vi "Kenbak-1.vi"() -> ()   [LabVIEW 2012]
uses:
  Blocks/NegJKflipFlop.vi
  <vilib>/Waveform/DTblOps.llb/DTbl Boolean Array to Digital.vi
panel:
  out "mem":u8 format="%x"
  in  "Set":bool
  in  "Oct":u8 format="%o"
  out "number":u32
  out "Array":bool[](array[boolean])
  in  "Loop":bool
  in  "Step 256":bool
  in  "Step 64":bool
  in  "Step 8":bool
  in  "Step 1":bool
  out "JS4":bool
  out "JS3":bool
  out "JS2":bool
  out "JS1":bool
  out "JS0":bool
  out "JDL1":bool
  out "JDL0":bool
  out "KP":bool
  out "PF":bool
  out "PT":bool
  out "PO":bool
  out "ED":bool
  out "WD":bool
  out "BM":bool
  out "WT":bool
  out "WL":bool
  out "WJ":bool
  out "WK":bool
  out "CY":bool
  out "OV":bool
  out "OF":bool
  out "CR":bool
  out "SUM":bool
  out "ADD":bool
  out "C":bool
  out "JC":bool
  out "TS":bool
  out "BD":bool
  out "B":bool
  out "A":bool
  out "LONGLOGIC":bool
  out "LS":bool
  out "RR":bool
  out "BT":bool
  out "TX":bool
  out "HF":bool
  out "JW3":bool
  out "JW7":bool
  out "W7":bool
  out "W6":bool
  out "W5":bool
  out "W4":bool
  out "W3":bool
  out "W2":bool
  out "W1":bool
  out "W0":bool
  out "K7":bool
  out "K6":bool
  out "K5":bool
  out "K4":bool
  out "K3":bool
  out "K2":bool
  out "K1":bool
  out "K0":bool
  out "KS":bool
  out "Run":bool
  out "Input":bool
  out "Mem":bool
  out "Add":bool
  out "X4":bool
  out "X3":bool
  out "X2":bool
  out "X1":bool
  out "BU":bool
  in  "S7":bool
  in  "S6":bool
  in  "S5":bool
  in  "S4":bool
  in  "S3":bool
  in  "S2":bool
  in  "S1":bool
  in  "S0":bool
  out "MR":bool
  out "FT":bool
  out "I4":bool
  out "I5":bool
  out "I6":bool
  out "I7":bool
  out "I3":bool
  out "I2":bool
  out "I1":bool
  out "I0":bool
  out "CL":bool
  out "DA":bool
  out "HT":bool
  out "EA":bool
  out "DD":bool
  out "EN":bool
  out "GO":bool
  out "UT":bool
  out "IN":bool
  in  "Clear":bool
  in  "Disp\nAdd":bool
  in  "Stop":bool
  in  "Set\nAdd":bool
  in  "Read\nMem":bool
  in  "Store\nMem":bool
  in  "Start":bool
  out "R":bool
  out "A7":bool
  out "SQ":bool
  out "SP":bool
  out "SW":bool
  out "SC":bool
  out "SD":bool
  out "SZ":bool
  out "SG":bool
  out "SM":bool
  out "SH":bool
  out "SK":bool
  out "SF":bool
  out "SN":bool
  out "SJ":bool
  out "SL":bool
  out "SA":bool
  out "QB":bool
  out "SX":bool
  out "SY":bool
  out "SB":bool
  out "ST":bool
  out "SV":bool
  out "SE":bool
  out "SU":bool
  out "SS":bool
  out "SR":bool
  out "QE":bool
  out "QF":bool
  out "QD":bool
  out "QC":bool
  in  "Plot?":bool
  out "Carry?":bool
  out "/ T7 \\":bool
  out "MemLoc":u8
  in  "Wait":u32=50
  in  "Diag?":bool
  out "LC":bool
  out "CM":bool
  out "L7":bool
  out "L6":bool
  out "L5":bool
  out "L4":bool
  out "L3":bool
  out "L2":bool
  out "L1":bool
  out "L0":bool
  out "Sigs":digitaldata(graph)
  out "T7":bool
  out "T6":bool
  out "T5":bool
  out "T4":bool
  out "T3":bool
  out "T2":bool
  out "T1":bool
  out "T0":bool
  out "F1":bool
  out "F2":bool
  out "C7":bool
  out "CP":bool
  out "CT":bool
  in  "Slices":u32=2
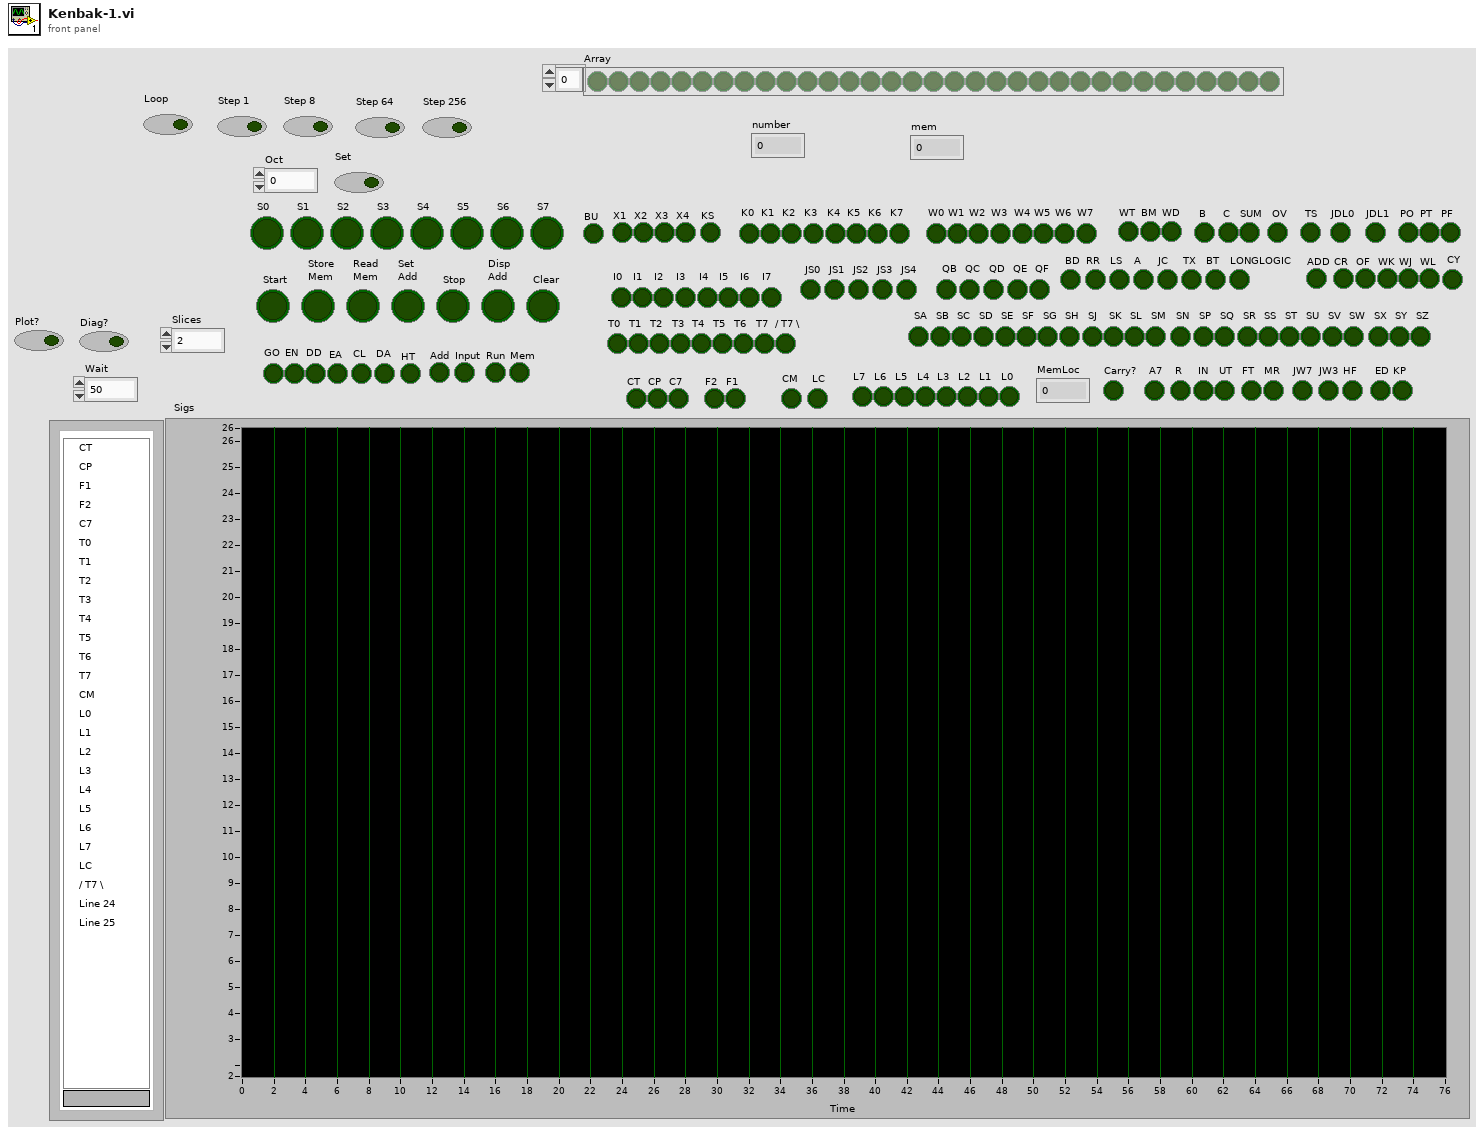
[diagram p1: front panel]
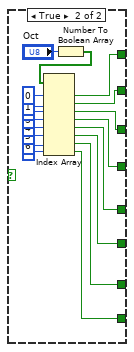
[diagram p2: hidden frame]
diagram:
  n1 = while {
    stop <- FALSE stop-if-true
    w68 = TRUE ("x")
    w107 = FALSE ("Serial\nInput")
    w149 = TRUE ("Set")
    w198 = TRUE ("Set")
    w199 = TRUE ("Set")
    w210 = FALSE ("y")
    w224 = TRUE ("Reset")
    w238 = TRUE ("Set")
    w249 = TRUE ("Set")
    w457 = TRUE ("Set")
    w458 = TRUE ("Set")
    w472 = TRUE ("Set")
    w605 = TRUE ("Set")
    w622 = TRUE ("Set")
    w629 = FALSE ("B")
    w630 = FALSE ("Mode\nControl")
    w633 = TRUE ("Set")
    w637 = FALSE ("B")
    w638 = FALSE ("Mode\nControl")
    w644 = TRUE
    w650 = TRUE ("Set")
    w652 = TRUE ("Set")
    # "JSX  0  1  2  3  4\nQB = 1, 0, 0, 1, 0\nQC = 0, 0, 0, 0, 0\nQD = 1, 0, 0, 0, 0\nQE = 1, 1, 0, 0, 0\nQF = 0, 1, 0, 0, 0\nSA = 0, 0, 0, 1, 0\nSB = 0, 0, 1, 1, 0\nSC = 0, 1, 0, 1, 1\nSD = 1, 1, 0, 1, 1\nSE = 1, 1, 1, 0, 0\nSF = 1, 1, 0, 0, 1\nSG = 1, 1, 1, 0, 1\nSH = 1, 0, 0, 0, 1\nSJ = 1, 0, 1, 0, 1\nSK = 0, 1, 0, 0, 1\nSL = 0, 1, 1, 0, 1\nSM = 0, 0, 0, 0, 1\nSN = 0, 0, 1, 0, 1\nSP = 0, 0, 0, 1, 1\nSQ = 0, 1, 1, 1, 1\nSR = 0, 0, 1, 0, 0\nSS = 1, 0, 1, 0, 0\nST = 1, 0, 1, 1, 0\nSU = 0, 1, 1, 0, 0\nSV = 0, 1, 1, 1, 0\nSW = 1, 0, 0, 1, 1\nSX = 0, 1, 0, 1, 0\nSY = 1, 1, 0, 1, 0\nSZ = 0, 0, 1, 1, 1"
    # "-IN+-BU"
    # "-IN+-CL"
    # "I11"
    # "I10"
    # "I2+-I1+I0"
    # "EN+DD"
    # "JS0"
    # "JS1"
    # "JS2"
    # "JS3"
    # "JS4"
    # "JS0B"
    # "JS0A"
    # "JS1B"
    # "JS2A"
    # "CM"
    # "JS1A"
    # "JS3A"
    # "JS3-4B"
    # "G5"
    # "G4"
    # "G3"
    # "G2"
    # "G1"
    n2 = call "Clock.vi"("Slices"="Slices") -> ("Clk"=w654:bool)  [unwired: 10 in]
    "CT" <- w654
    n3 = case shown="False" "Set" {
      tunnel: ["S0" w678] -> w44
      tunnel: ["S1" w669] -> w43
      tunnel: ["S2" w668] -> w41
      tunnel: ["S3" w667] -> w39
      tunnel: ["S4" w666] -> w37
      tunnel: ["S5" w665] -> w35
      tunnel: ["S6" w664] -> w33
      tunnel: ["S7" w663] -> w30
      frame False {
      }
      frame True {
        n4 = Number To Boolean Array(number="Oct") -> (Boolean array=w679:bool[])
        n5 = Index Array(array=w679, index #1=0 ("index"), index #2=1 ("index"), index #3=2 ("index"), index #4=3 ("index"), index #5=4 ("index"), index #6=5 ("index"), index #7=6 ("index"), index #8=7 ("index")) -> (element #1=w678:bool, element #2=w669:bool, element #3=w668:bool, element #4=w667:bool, element #5=w666:bool, element #6=w665:bool, element #7=w664:bool, element #8=w663:bool)
      }
    }
    n6 = Not And(1:w654, 2:w654) -> (0:w653:bool)
    n7 = feedback #1() -> (w651:bool)  [unwired: 1 in]
    n8 = call "DflipFlop.vi"("D"=w651, "Clock"=w653, "Reset"=w652, "Set"=w652) -> ("/Q\\"=w27:bool, "Q"=w639:bool)  [unwired: 6 in]
    n9 = feedback-in #1(w27) -> ()
    n10 = Not(x=w35) -> (.not. x?=w34:bool)
    n11 = Not(x=w33) -> (.not. x?=w32:bool)
    n12 = Not(x=w30) -> (.not. x?=w31:bool)
    n13 = Not(x=w44) -> (.not. x?=w45:bool)
    n14 = Not(x=w43) -> (.not. x?=w42:bool)
    n15 = Not(x=w41) -> (.not. x?=w40:bool)
    n16 = Not(x=w39) -> (.not. x?=w38:bool)
    n17 = Not(x=w37) -> (.not. x?=w36:bool)
    n18 = feedback #2() -> (w607:bool)  [unwired: 1 in]
    n19 = Not(x="Stop") -> (.not. x?=w4:bool)
    "HT" <- w4
    n20 = Not(x="Start") -> (.not. x?=w464:bool)
    n21 = Not(x="Read\nMem") -> (.not. x?=w462:bool)
    n22 = Not(x="Set\nAdd") -> (.not. x?=w461:bool)
    n23 = Not(x="Disp\nAdd") -> (.not. x?=w392:bool)
    "DA" <- w392
    n24 = Not(x="Clear") -> (.not. x?=w80:bool)
    "CL" <- w80
    n25 = Not(x="Store\nMem") -> (.not. x?=w463:bool)
    n26 = feedback #3() -> (w647:bool)  [unwired: 1 in]
    n27 = Compound Arithmetic op=AND(w647, w647, w607) -> (w649:bool)
    n28 = Not(x=w649) -> (.not. x?=w648:bool)
    n29 = call "DflipFlop.vi"("D"=w648, "Clock"=w639, "Reset"=w650, "Set"=w650) -> ("/Q\\"=w643:bool, "Q"=w642:bool)  [unwired: 6 in]
    n30 = feedback-in #3(w642) -> ()
    n31 = Not And(1:w639, 2:w639) -> (0:w641:bool)
    n32 = feedback #4() -> (w635:bool)  [unwired: 1 in]
    n33 = Not And(1:w635, 2:w639) -> (0:w640:bool)
    n34 = Not And(1:w635, 2:w635) -> (0:w606:bool)
    "/ T7 \\" <- w606
    n35 = feedback-in #2(w606) -> ()
    n36 = Not(x=w641) -> (.not. x?=w106:bool)
    "CP" <- w106
    n37 = call "7495.vi"("Clk 1\nR-Shift"=w106, "Serial\nInput"=w635, "Clk 2\nL-Shift"=w106, "Mode\nControl"=w638, "D"=w638, "C"=w638, "B"=w638, "A"=w638) -> ("OD"=w409:bool, "OC"=w410:bool, "OB"=w85:bool, "OA"=w87:bool)
    "T0" <- w87
    "T1" <- w85
    "T2" <- w410
    "T3" <- w409
    n38 = Not And(1:w45, 2:w87) -> (0:w406:bool)
    n39 = Not And(1:w42, 2:w85) -> (0:w405:bool)
    n40 = Not And(1:w40, 2:w410) -> (0:w404:bool)
    n41 = Not And(1:w38, 2:w409) -> (0:w403:bool)
    n42 = Not(x=w640) -> (.not. x?=w234:bool)
    "C7" <- w234
    n43 = Not And(1:w234, 2:w234) -> (0:w513:bool)
    n44 = call "7495.vi"("Clk 1\nR-Shift"=w106, "Serial\nInput"=FALSE ("Serial\nInput"), "Clk 2\nL-Shift"=w106, "Mode\nControl"=w409, "D"=w637, "C"=w637, "B"=w637, "A"=w409) -> ("OD"=w14:bool, "OC"=w407:bool, "OB"=w408:bool, "OA"=w296:bool)
    "T4" <- w296
    "T5" <- w408
    "T6" <- w407
    "T7" <- w14
    n45 = feedback-in #4(w14) -> ()
    n46 = Not And(1:w36, 2:w296) -> (0:w402:bool)
    n47 = Not And(1:w234, 2:w234) -> (0:w456:bool)
    n48 = feedback #5() -> (w394:bool)  [unwired: 1 in]
    n49 = feedback #6() -> (w393:bool)  [unwired: 1 in]
    n50 = Not And(1:w34, 2:w408) -> (0:w401:bool)
    n51 = Compound Arithmetic op=AND(w643, w644, w27) -> (w645:bool)
    n52 = Compound Arithmetic op=AND(w644, w27, w642) -> (w646:bool)
    n53 = Not(x=w645) -> (.not. x?=w73:bool)
    "F1" <- w73
    n54 = Not(x=w646) -> (.not. x?=w71:bool)
    "F2" <- w71
    n55 = feedback #7() -> (w455:bool)  [unwired: 1 in]
    n56 = call "DflipFlop.vi"("D"=w455, "Clock"=w456, "Reset"=w458, "Set"=w458) -> ("Q"=w378:bool)  [unwired: 6 in, 1 out]
    "UT" <- w378
    n57 = Not And(1:w32, 2:w407) -> (0:w400:bool)
    n58 = Exclusive Or(1:w106, 2:TRUE ("x")) -> (0:w621:bool)
    n59 = Not And(1:w31, 2:w14) -> (0:w399:bool)
    n60 = Compound Arithmetic op=AND(w80, w80, w80) -> (w82:bool)
    n61 = Not(x=w82) -> (.not. x?=w81:bool)
    n62 = Compound Arithmetic op=AND(w406, w405, w404, w403, w402, w401, w400, w399) -> (w25:bool)
    "BU" <- w25
    n63 = Not And(1:w25, 2:w25) -> (0:w26:bool)
    n64 = feedback #8() -> (w627:bool)  [unwired: 1 in]
    n65 = feedback #9() -> (w619:bool)  [unwired: 1 in]
    n66 = Not And(1:w619, 2:w627) -> (0:w632:bool)
    n67 = Not And(1:w606, 2:w632) -> (0:w631:bool)
    n68 = Exclusive Or(1:w619, 2:w627) -> (0:w628:bool)
    n69 = call "7495.vi"("Clk 1\nR-Shift"=w106, "Serial\nInput"=w628, "Clk 2\nL-Shift"=w106, "Mode\nControl"=w630, "D"=w630, "C"=w630, "A"=w619) -> ("OD"=w612:bool, "OC"=→"L5":bool, "OB"=→"L6":bool, "OA"=→"L7":bool)  [unwired: 1 in]
    "L4" <- w612
    n70 = call "DflipFlop.vi"("D"=w631, "Clock"=w621, "Reset"=w633, "Set"=w633) -> ("Q"=w451:bool)  [unwired: 6 in, 1 out]
    "LC" <- w451
    n71 = call "DflipFlop.vi"("D"=w451, "Clock"=w456, "Reset"=w457, "Set"=w457) -> ("Q"=w78:bool)  [unwired: 6 in, 1 out]
    "IN" <- w78
    n72 = call "7495.vi"("Clk 1\nR-Shift"=w78, "Serial\nInput"=FALSE ("Serial\nInput"), "Clk 2\nL-Shift"=w78, "Mode\nControl"=TRUE ("Mode\nControl"), "D"=w461, "C"=w462, "B"=w463, "A"=w464) -> ("OD"=w342:bool, "OC"=w390:bool, "OB"=w178:bool, "OA"=w51:bool)
    "GO" <- w51
    "EN" <- w178
    "DD" <- w390
    "EA" <- w342
    n73 = Not And(1:w51, 2:w51) -> (0:w50:bool)
    n74 = Compound Arithmetic op=AND(w392, w390, w394) -> (w397:bool)
    n75 = Compound Arithmetic op=AND(w178, w390, w392, w392) -> (w454:bool)
    n76 = Compound Arithmetic op=AND(w178, w390, w390, w178) -> (w453:bool)
    n77 = Not(x=w397) -> (.not. x?=w389:bool)
    n78 = Not(x=w454) -> (.not. x?=w452:bool)
    n79 = Not(x=w453) -> (.not. x?=w262:bool)
    n80 = feedback-in #7(w78) -> ()
    n81 = Not And(1:w81, 2:w78) -> (0:w79:bool)
    n82 = Not And(1:w25, 2:w78) -> (0:w77:bool)
    n83 = feedback-in #8(w451) -> ()
    n84 = And(x=w14, y=w451) -> (x .and. y?=→"Carry?":bool)
    n85 = Not And(1:w342, 2:w342) -> (0:w343:bool)
    n86 = call "7495.vi"("Clk 1\nR-Shift"=w106, "Serial\nInput"=w612, "Clk 2\nL-Shift"=w106, "Mode\nControl"=w629, "D"=w106, "C"=w619, "B"=w629, "A"=w629) -> ("OD"=w616:bool, "OC"=→"L1":bool, "OB"=→"L2":bool, "OA"=→"L3":bool)
    "L0" <- w616
    n87 = feedback-in #9(w616) -> ()
    n88 = feedback #10() -> (w370:bool)  [unwired: 1 in]
    n89 = feedback #11() -> (w371:bool)  [unwired: 1 in]
    n90 = feedback #12() -> (w372:bool)  [unwired: 1 in]
    n91 = feedback #13() -> (w373:bool)  [unwired: 1 in]
    n92 = feedback #14() -> (w626:bool)  [unwired: 1 in]
    n93 = feedback #15() -> (w443:bool)  [unwired: 1 in]
    n94 = feedback #16() -> (w444:bool)  [unwired: 1 in]
    n95 = feedback #17() -> (w445:bool)  [unwired: 1 in]
    n96 = feedback #18() -> (w446:bool)  [unwired: 1 in]
    n97 = feedback #19() -> (w377:bool)  [unwired: 1 in]
    n98 = feedback #20() -> (w376:bool)  [unwired: 1 in]
    n99 = feedback #21() -> (w375:bool)  [unwired: 1 in]
    n100 = feedback #22() -> (w374:bool)  [unwired: 1 in]
    n101 = feedback #23() -> (w450:bool)  [unwired: 1 in]
    n102 = feedback #24() -> (w449:bool)  [unwired: 1 in]
    n103 = feedback #25() -> (w448:bool)  [unwired: 1 in]
    n104 = feedback #26() -> (w447:bool)  [unwired: 1 in]
    n105 = Not And(1:w87, 2:w87) -> (0:w298:bool)
    n106 = Not And(1:w296, 2:w296) -> (0:w285:bool)
    n107 = feedback #27() -> (w300:bool)  [unwired: 1 in]
    n108 = feedback #28() -> (w512:bool)  [unwired: 1 in]
    n109 = call "DflipFlop.vi"("D"=w512, "Clock"=w513, "Reset"=w605, "Set"=w605) -> ("Q"=w600:bool)  [unwired: 6 in, 1 out]
    "JS0" <- w600
    n110 = feedback #29() -> (w511:bool)  [unwired: 1 in]
    n111 = call "DflipFlop.vi"("D"=w511, "Clock"=w513, "Reset"=w605, "Set"=w605) -> ("Q"=w599:bool)  [unwired: 6 in, 1 out]
    "JS1" <- w599
    n112 = feedback #30() -> (w510:bool)  [unwired: 1 in]
    n113 = call "DflipFlop.vi"("D"=w510, "Clock"=w513, "Reset"=w605, "Set"=w605) -> ("Q"=w598:bool)  [unwired: 6 in, 1 out]
    "JS2" <- w598
    n114 = feedback #31() -> (w509:bool)  [unwired: 1 in]
    n115 = call "DflipFlop.vi"("D"=w509, "Clock"=w513, "Reset"=w605, "Set"=w605) -> ("/Q\\"=w601:bool, "Q"=w603:bool)  [unwired: 6 in]
    "JS3" <- w603
    n116 = feedback #32() -> (w508:bool)  [unwired: 1 in]
    n117 = call "DflipFlop.vi"("D"=w508, "Clock"=w513, "Reset"=w605, "Set"=w605) -> ("/Q\\"=w604:bool, "Q"=w602:bool)  [unwired: 6 in]
    "JS4" <- w602
    n118 = Not And(1:w604, 2:w601) -> (0:w594:bool)
    n119 = Not And(1:w604, 2:w603) -> (0:w595:bool)
    n120 = Not And(1:w602, 2:w601) -> (0:w596:bool)
    n121 = Not And(1:w602, 2:w603) -> (0:w597:bool)
    n122 = call "7442.vi"("D"=w597, "C"=w598, "B"=w599, "A"=w600) -> ("0"=w440:bool, "1"=w326:bool, "2"=w482:bool, "3"=w138:bool, "4"=w536:bool, "6"=w109:bool)  [unwired: 2 in, 4 out]
    "SP" <- w440
    "SW" <- w326
    "SC" <- w482
    "SD" <- w138
    "SZ" <- w536
    "SQ" <- w109
    n123 = call "7442.vi"("D"=w594, "C"=w598, "B"=w599, "A"=w600) -> ("0"=w48:bool, "1"=w480:bool, "2"=w572:bool, "3"=w177:bool, "4"=w479:bool, "5"=w179:bool, "6"=w110:bool, "7"=w116:bool)  [unwired: 2 in, 2 out]
    "QC" <- w48
    "QD" <- w480
    "QF" <- w572
    "QE" <- w177
    "SR" <- w479
    "SS" <- w179
    "SU" <- w110
    "SE" <- w116
    "Run" <- w48
    n124 = call "7442.vi"("D"=w595, "C"=w598, "B"=w599, "A"=w600) -> ("0"=w391:bool, "1"=w533:bool, "2"=w519:bool, "3"=w187:bool, "4"=w104:bool, "5"=w485:bool, "6"=w346:bool)  [unwired: 2 in, 3 out]
    "SA" <- w391
    "QB" <- w533
    "SX" <- w519
    "SY" <- w187
    "SB" <- w104
    "ST" <- w485
    "SV" <- w346
    n125 = Compound Arithmetic op=AND(w389, w391, w80, w26) -> (w398:bool)
    n126 = Compound Arithmetic op=AND(w392, w391, w393) -> (w396:bool)
    n127 = Not(x=w398) -> (.not. x?=w387:bool)
    n128 = feedback-in #5(w387) -> ()
    n129 = Not(x=w396) -> (.not. x?=w388:bool)
    n130 = Compound Arithmetic op=AND(w388, w390, w80, w26) -> (w395:bool)
    n131 = Not(x=w395) -> (.not. x?=w386:bool)
    n132 = feedback-in #6(w386) -> ()
    n133 = And(x=w388, y=w389) -> (x .and. y?=w46:bool)
    "X1" <- w46
    "Add" <- w46
    n134 = And(x=w389, y=w386) -> (x .and. y?=w47:bool)
    "X2" <- w47
    "Mem" <- w47
    n135 = And(x=w388, y=w387) -> (x .and. y?=w362:bool)
    "X3" <- w362
    n136 = And(x=w387, y=w386) -> (x .and. y?=w49:bool)
    "X4" <- w49
    "Input" <- w49
    n137 = call "7442.vi"("D"=w596, "C"=w598, "B"=w599, "A"=w600) -> ("0"=w55:bool, "1"=w486:bool, "2"=w478:bool, "3"=w481:bool, "4"=w268:bool, "5"=w257:bool, "6"=w347:bool, "7"=w53:bool)  [unwired: 2 in, 2 out]
    "SM" <- w55
    "SH" <- w486
    "SK" <- w478
    "SF" <- w481
    "SN" <- w268
    "SJ" <- w257
    "SL" <- w347
    "SG" <- w53
    n138 = Not And(1:w177, 2:w177) -> (0:w379:bool)
    n139 = And(x=w379, y=w47) -> (x .and. y?=w380:bool)
    n140 = And(x=w379, y=w46) -> (x .and. y?=w381:bool)
    n141 = And(x=w78, y=w49) -> (x .and. y?=w382:bool)
    n142 = And(x=w362, y=w378) -> (x .and. y?=w383:bool)
    n143 = Compound Arithmetic op=OR(w380, w381, w382, w383) -> (w384:bool)
    n144 = Not(x=w384) -> (.not. x?=w369:bool)
    "KS" <- w369
    n145 = Not And(1:w48, 2:w48) -> (0:w441:bool)
    n146 = Not And(1:w78, 2:w441) -> (0:w345:bool)
    n147 = Not And(1:w345, 2:w345) -> (0:w344:bool)
    n148 = Compound Arithmetic op=AND(w138, w109, w177, w179, w345, w345, w440, w177) -> (w442:bool)
    n149 = Not(x=w442) -> (.not. x?=w12:bool)
    "FT" <- w12
    n150 = Not And(1:w343, 2:w344) -> (0:w341:bool)
    n151 = Not And(1:w12, 2:w12) -> (0:w13:bool)
    n152 = Not(x=w55) -> (.not. x?=w54:bool)
    n153 = Not(x=w480) -> (.not. x?=w573:bool)
    n154 = Not(x=w104) -> (.not. x?=w592:bool)
    n155 = Not(x=w485) -> (.not. x?=w56:bool)
    n156 = Not(x=w347) -> (.not. x?=w158:bool)
    n157 = Not And(1:w116, 2:w116) -> (0:w264:bool)
    n158 = Not And(1:w572, 2:w572) -> (0:w571:bool)
    n159 = Not And(1:w53, 2:w53) -> (0:w52:bool)
    n160 = Not And(1:w48, 2:w48) -> (0:w502:bool)
    n161 = Not And(1:w536, 2:w536) -> (0:w585:bool)
    n162 = Not And(1:w346, 2:w346) -> (0:w145:bool)
    n163 = Compound Arithmetic op=AND(w138, w138, w110, w110) -> (w590:bool)
    n164 = Not(x=w590) -> (.not. x?=w589:bool)
    n165 = Not And(1:w589, 2:w589) -> (0:w523:bool)
    n166 = Not And(1:w110, 2:w519) -> (0:w490:bool)
    n167 = And(x=w50, y=w502) -> (x .and. y?=w583:bool)
    n168 = Not And(1:w55, 2:w55) -> (0:w487:bool)
    n169 = feedback #33() -> (w297:bool)  [unwired: 1 in]
    n170 = Not And(1:w297, 2:w298) -> (0:w295:bool)
    n171 = Not And(1:w285, 2:w295) -> (0:w294:bool)
    n172 = feedback-in #33(w294) -> ()
    n173 = feedback #34() -> (w306:bool)  [unwired: 1 in]
    n174 = And(x=w571, y=w452) -> (x .and. y?=w576:bool)
    n175 = Compound Arithmetic op=AND(w257, w55, w116, w53) -> (w544:bool)
    n176 = Compound Arithmetic op=AND(w138, w482, w481, w480, w479, w478, w478, w479) -> (w492:bool)
    n177 = Not(x=w544) -> (.not. x?=w543:bool)
    n178 = Not(x=w492) -> (.not. x?=w475:bool)
    n179 = Not And(1:w326, 2:w326) -> (0:w319:bool)
    n180 = Not And(1:w543, 2:w543) -> (0:w545:bool)
    n181 = Not And(1:w48, 2:w48) -> (0:w474:bool)
    n182 = And(x=w48, y=FALSE) -> (x .and. y?=w499:bool)
    n183 = Compound Arithmetic op=AND(w177, w116, w104, w53, w347, w346, w341, w257) -> (w348:bool)
    n184 = Not And(1:w138, 2:w138) -> (0:w139:bool)
    n185 = while {
      tunnel: "Slices" -> [w682]
      stop <- w704 stop-if-true
      n186 = Multiply(x=w682, y=u32 64 ("Delay")) -> (x*y=w687:u32)
      n187 = Multiply(x=w682, y=u32 256 ("Delay")) -> (x*y=w688:u32)
      n188 = Multiply(x=w682, y=u32 8 ("Delay")) -> (x*y=w685:u32)
      n189 = Multiply(x=w682, y=u32 1 ("Delay")) -> (x*y=w683:u32)
      n190 = call "TriggerDelay.vi"("Delay"=w688, "In"="Step 256") -> ("Off"=w693:bool, "Out"=w697:bool)  [unwired: 8 in]
      n191 = call "TriggerDelay.vi"("Delay"=w687, "In"="Step 64") -> ("Off"=w692:bool, "Out"=w698:bool)  [unwired: 8 in]
      n192 = call "TriggerDelay.vi"("Delay"=w685, "In"="Step 8") -> ("Off"=w691:bool, "Out"=w695:bool)  [unwired: 8 in]
      n193 = call "TriggerDelay.vi"("Delay"=w683, "In"="Step 1") -> ("Off"=w690:bool, "Out"=w696:bool)  [unwired: 8 in]
      n194 = Compound Arithmetic op=OR(w697, w698, w695, w696, "Loop") -> (w704:bool)
      n195 = Compound Arithmetic op=OR(w693, w692, w691, w690) -> (w694:bool)
      n196 = case shown="True" w694 {
        frame False {
        }
        frame True {
          w705 = FALSE
          n197 = local write "Step 256"(w705) -> ()
          n198 = local write "Step 64"(w705) -> ()
          n199 = local write "Step 1"(w705) -> ()
          n200 = local write "Step 8"(w705) -> ()
        }
      }
    }
    n201 = Not And(1:w533, 2:w533) -> (0:w554:bool)
    n202 = And(x=w474, y=w474) -> (x .and. y?=w477:bool)
    n203 = Not(x=w348) -> (.not. x?=w334:bool)
    n204 = feedback #35() -> (w287:bool)  [unwired: 1 in]
    n205 = And(x=w554, y=w50) -> (x .and. y?=w555:bool)
    n206 = And(x=w502, y=w452) -> (x .and. y?=w558:bool)
    n207 = Not And(1:w50, 2:w502) -> (0:w551:bool)
    n208 = Not And(1:w334, 2:w334) -> (0:w337:bool)
    n209 = Compound Arithmetic op=AND(w179, w187, w346, w268, w268, w536, w536, w536) -> (w539:bool)
    n210 = Not(x=w539) -> (.not. x?=w538:bool)
    n211 = Not And(1:w106, 2:w106) -> (0:w220:bool)
    n212 = Not And(1:w14, 2:w14) -> (0:w223:bool)
    n213 = Not And(1:w538, 2:w538) -> (0:w537:bool)
    n214 = Not And(1:w234, 2:w234) -> (0:w197:bool)
    n215 = Compound Arithmetic op=AND(w486, w478, w481, w391) -> (w531:bool)
    n216 = Not(x=w531) -> (.not. x?=w530:bool)
    n217 = feedback #36() -> (w246:bool)  [unwired: 1 in]
    n218 = Compound Arithmetic op=AND(w479, w519, w482, w482) -> (w501:bool)
    n219 = Not(x=w501) -> (.not. x?=w520:bool)
    n220 = feedback #37() -> (w313:bool)  [unwired: 1 in]
    n221 = feedback #38() -> (w356:bool)  [unwired: 1 in]
    n222 = feedback #39() -> (w357:bool)  [unwired: 1 in]
    n223 = feedback #40() -> (w314:bool)  [unwired: 1 in]
    n224 = Not And(1:w177, 2:w177) -> (0:w263:bool)
    n225 = feedback #41() -> (w360:bool)  [unwired: 1 in]
    n226 = feedback #42() -> (w359:bool)  [unwired: 1 in]
    n227 = feedback #43() -> (w358:bool)  [unwired: 1 in]
    n228 = feedback #44() -> (w312:bool)  [unwired: 1 in]
    n229 = And(x=w46, y=w312) -> (x .and. y?=w368:bool)
    n230 = And(x=w312, y=w475) -> (x .and. y?=w484:bool)
    n231 = And(x=w475, y=w312) -> (x .and. y?=w476:bool)
    n232 = Not Or(1:w477, 2:w476) -> (0:w473:bool)
    n233 = call "DflipFlop.vi"("D"=w473, "Clock"=w234, "Reset"=w472, "Set"=w472) -> ("/Q\\"=w11:bool, "Q"=w10:bool)  [unwired: 6 in]
    "A7" <- w11
    n234 = Not And(1:w116, 2:w116) -> (0:w265:bool)
    n235 = Not And(1:w268, 2:w268) -> (0:w182:bool)
    n236 = Not And(1:w262, 2:w263) -> (0:w259:bool)
    n237 = Not And(1:w104, 2:w104) -> (0:w252:bool)
    n238 = Not And(1:w109, 2:w109) -> (0:w250:bool)
    n239 = Not And(1:w14, 2:w14) -> (0:w222:bool)
    n240 = Wait (ms)(milliseconds to wait="Wait") -> ()  [unwired: 1 out]
    n241 = And(x=w85, y=w250) -> (x .and. y?=w271:bool)
    n242 = Not And(1:w4, 2:w4) -> (0:w5:bool)
    n243 = Not And(1:w109, 2:w187) -> (0:w186:bool)
    n244 = Not And(1:w178, 2:w178) -> (0:w176:bool)
    n245 = Not And(1:w177, 2:w177) -> (0:w175:bool)
    n246 = case shown="True" "Diag?" {
      frame False {
      }
      frame True {
        n247 = local read "CT"() -> (w713:bool)
        n248 = local read "CP"() -> (w712:bool)
        n249 = local read "F1"() -> (w714:bool)
        n250 = local read "F2"() -> (w738:bool)
        n251 = local read "C7"() -> (w709:bool)
        n252 = local read "T0"() -> (w707:bool)
        n253 = local read "T1"() -> (w706:bool)
        n254 = local read "T6"() -> (w733:bool)
        n255 = local read "T7"() -> (w732:bool)
        n256 = local read "T2"() -> (w737:bool)
        n257 = local read "T4"() -> (w735:bool)
        n258 = local read "T5"() -> (w734:bool)
        n259 = local read "T3"() -> (w736:bool)
        n260 = Build Array(w713, w712, w714, w738, w709, w707, w706, w737, w736, w735, w734, w733, w732) -> (w725:bool[])
        n261 = local read "/ T7 \\"() -> (w729:bool)
        n262 = local read "CM"() -> (w726:bool)
        n263 = local read "CP"() -> (w730:bool)
        n264 = local read "CP"() -> (w731:bool)
        n265 = local read "L0"() -> (w727:bool)
        n266 = local read "L1"() -> (w722:bool)
        n267 = local read "L2"() -> (w721:bool)
        n268 = local read "L4"() -> (w719:bool)
        n269 = local read "L5"() -> (w718:bool)
        n270 = local read "LC"() -> (w728:bool)
        n271 = local read "L3"() -> (w720:bool)
        n272 = local read "L6"() -> (w717:bool)
        n273 = local read "L7"() -> (w716:bool)
        n274 = And(x=w713, y=w712) -> (x .and. y?=w710:bool)
        n275 = Build Array(w726, w727, w722, w721, w720, w719, w718, w717, w716, w728, w729, w730, w731) -> (w724:bool[])
        n276 = Build Array (concatenate)(w725, w724) -> (w723:bool[])
        n277 = case shown="True" "Plot?" {
          tunnel: w723 -> [_ w751]
          frame False {
          }
          frame True {
            n278 = feedback #45(bool[][] []) -> (w753:bool[][])
            n279 = Build Array (concatenate)(w753, w751) -> (w755:bool[][])
            n280 = feedback-in #45(w755) -> ()
            n281 = call-poly <vilib>:"Boolean Array to Digital.vi"("boolean array"=w753) -> ("digital data"=→"Sigs":digitaldata)  [unwired: 9 in, 1 out]
          }
        }
        n282 = feedback #46() -> (w711:bool)  [unwired: 1 in]
        n283 = feedback-in #46(w710) -> ()
        n284 = case shown="True" w709 {
          tunnel: w722 -> [_ w762]
          tunnel: w721 -> [_ w761]
          tunnel: w720 -> [_ w760]
          tunnel: w719 -> [_ w759]
          tunnel: w718 -> [_ w758]
          tunnel: w717 -> [_ w757]
          tunnel: w716 -> [_ w756]
          frame False {
          }
          frame True {
            n285 = Build Array(w762, w761, w760, w759, w758, w757, w756) -> (w763:bool[])
            n286 = Boolean Array To Number(Boolean array=w763) -> (number=→"MemLoc":u32)
          }
        }
        n287 = Less?(x=w710, y=w711) -> (x < y?=w708:bool)
        n288 = case shown="True" w708 {
          tunnel: w706 -> [_ w741]
          frame False {
          }
          frame True {
            n289 = local read "Array"() -> (w748:bool[])
            n290 = local read "R"() -> (w747:bool)
            n291 = Not(x=w747) -> (.not. x?=w740:bool)
            n292 = Build Array(w740) -> (w739:bool[])
            n293 = Build Array (concatenate)(w748, w740) -> (w743:bool[])
            n294 = Select(t=w739, s=w741, f=w743) -> (s? t:f=w742:bool[])
            "Array" <- w742
            n295 = Array Size(array=w742) -> (size(s)=w746:i32)
            n296 = Equal?(x=w746, y=8) -> (x = y?=w744:bool)
            n297 = case shown="True" w744 {
              tunnel: w742 -> [_ w750]
              frame False {
              }
              frame True {
                n298 = Boolean Array To Number(Boolean array=w750) -> (number=→"number":u32)
              }
            }
          }
        }
      }
    }
    n299 = Not And(1:w186, 2:w186) -> (0:w183:bool)
    n300 = Not And(1:w176, 2:w175) -> (0:w174:bool)
    n301 = Not And(1:w174, 2:w179) -> (0:w152:bool)
    "WL" <- w152
    n302 = And(x=w152, y=w152) -> (x .and. y?=w171:bool)
    n303 = Not And(1:TRUE ("y"), 2:w106) -> (0:w135:bool)
    n304 = feedback #47() -> (w216:bool)  [unwired: 1 in]
    n305 = call "7495.vi"("Clk 1\nR-Shift"=w106, "Serial\nInput"=w216, "Clk 2\nL-Shift"=w106, "Mode\nControl"=w13, "D"=w446, "C"=w445, "B"=w444, "A"=w443) -> ("OD"=w194:bool, "OC"=w292:bool, "OB"=w155:bool, "OA"=w124:bool)
    "I4" <- w194
    "I5" <- w292
    "I6" <- w155
    "I7" <- w124
    n306 = feedback-in #15(w124) -> ()
    n307 = feedback-in #16(w155) -> ()
    n308 = feedback-in #17(w292) -> ()
    n309 = feedback-in #18(w194) -> ()
    n310 = call "7495.vi"("Clk 1\nR-Shift"=w106, "Serial\nInput"=w194, "Clk 2\nL-Shift"=w106, "Mode\nControl"=w13, "D"=w447, "C"=w448, "B"=w449, "A"=w450) -> ("OD"=w143:bool, "OC"=w227:bool, "OB"=w424:bool, "OA"=w190:bool)
    "I0" <- w143
    "I1" <- w227
    "I2" <- w424
    "I3" <- w190
    n311 = feedback-in #23(w190) -> ()
    n312 = feedback-in #24(w424) -> ()
    n313 = feedback-in #25(w227) -> ()
    n314 = feedback-in #26(w143) -> ()
    n315 = Not(x=w292) -> (.not. x?=w181:bool)
    n316 = Not And(1:w194, 2:w194) -> (0:w434:bool)
    n317 = Not(x=w143) -> (.not. x?=w427:bool)
    n318 = Not And(1:w424, 2:w424) -> (0:w426:bool)
    n319 = Compound Arithmetic op=AND(w426, w427, w227) -> (w433:bool)
    n320 = Not And(1:w143, 2:w145) -> (0:w515:bool)
    n321 = Not(x=w433) -> (.not. x?=w163:bool)
    n322 = Not And(1:w158, 2:w163) -> (0:w542:bool)
    n323 = Not And(1:w158, 2:w542) -> (0:w534:bool)
    n324 = Not And(1:w227, 2:w227) -> (0:w422:bool)
    n325 = Not And(1:w143, 2:w143) -> (0:w421:bool)
    n326 = Not(x=w155) -> (.not. x?=w126:bool)
    n327 = Not And(1:w155, 2:w124) -> (0:w280:bool)
    n328 = Not And(1:w190, 2:w194) -> (0:w308:bool)
    n329 = Not And(1:w124, 2:w124) -> (0:w162:bool)
    n330 = Not And(1:w181, 2:w181) -> (0:w428:bool)
    n331 = Not And(1:w421, 2:w422) -> (0:w423:bool)
    n332 = Not(x=w280) -> (.not. x?=w437:bool)
    n333 = Not(x=w280) -> (.not. x?=w191:bool)
    n334 = Not And(1:w424, 2:w424) -> (0:w279:bool)
    n335 = Not And(1:w190, 2:w190) -> (0:w307:bool)
    n336 = Not And(1:w437, 2:w308) -> (0:w261:bool)
    n337 = Not(x=w308) -> (.not. x?=w436:bool)
    n338 = Compound Arithmetic op=AND(w181, w143, w424) -> (w430:bool)
    n339 = Compound Arithmetic op=AND(w423, w181, w424) -> (w425:bool)
    n340 = Compound Arithmetic op=AND(w163, w428, w190) -> (w429:bool)
    n341 = Not And(1:w307, 2:w279) -> (0:w435:bool)
    n342 = Not And(1:w190, 2:w194) -> (0:w232:bool)
    n343 = Not And(1:w307, 2:w194) -> (0:w311:bool)
    n344 = Not And(1:w190, 2:w308) -> (0:w310:bool)
    n345 = Not And(1:w307, 2:w308) -> (0:w309:bool)
    n346 = Not And(1:w280, 2:w124) -> (0:w438:bool)
    n347 = Not And(1:w155, 2:w280) -> (0:w439:bool)
    n348 = Not(x=w430) -> (.not. x?=w417:bool)
    n349 = Not(x=w425) -> (.not. x?=w414:bool)
    n350 = Not(x=w429) -> (.not. x?=w416:bool)
    n351 = Not And(1:w436, 2:w280) -> (0:w431:bool)
    n352 = Not And(1:w431, 2:w181) -> (0:w564:bool)
    n353 = Compound Arithmetic op=AND(w431, w422, w181, w424) -> (w432:bool)
    n354 = Not(x=w432) -> (.not. x?=w418:bool)
    n355 = Not(x=w438) -> ()  [unwired: 1 out]
    n356 = Not(x=w439) -> (.not. x?=w413:bool)
    n357 = Not And(1:w431, 2:w431) -> (0:w7:bool)
    n358 = Not And(1:w7, 2:w181) -> (0:w503:bool)
    n359 = call "7495.vi"("Clk 1\nR-Shift"=w106, "Serial\nInput"=w306, "Clk 2\nL-Shift"=w106, "Mode\nControl"=w14, "D"=w309, "C"=w310, "B"=w311, "A"=w232) -> ("OD"=w293:bool)  [unwired: 3 out]
    "TX" <- w293
    n360 = Compound Arithmetic op=AND(w418, w163, w417, w416) -> (w419:bool)
    n361 = Not(x=w181) -> (.not. x?=w420:bool)
    n362 = Not And(1:w414, 2:w416) -> (0:w6:bool)
    n363 = Not(x=w419) -> (.not. x?=w415:bool)
    n364 = feedback-in #34(w293) -> ()
    n365 = Compound Arithmetic op=AND(w52, w181, w422) -> (w561:bool)
    n366 = Not And(1:w293, 2:w293) -> (0:w288:bool)
    n367 = Compound Arithmetic op=AND(w288, w298, w288) -> (w305:bool)
    n368 = Not(x=w305) -> (.not. x?=w301:bool)
    n369 = Not And(1:w300, 2:w301) -> (0:w283:bool)
    "RR" <- w283
    n370 = Not And(1:w298, 2:w283) -> (0:w299:bool)
    n371 = feedback-in #27(w299) -> ()
    n372 = Not And(1:w292, 2:w292) -> (0:w233:bool)
    n373 = Not And(1:w487, 2:w413) -> (0:w489:bool)
    n374 = Not And(1:w420, 2:w490) -> (0:w491:bool)
    n375 = Not And(1:w413, 2:w487) -> (0:w488:bool)
    n376 = Not(x=w561) -> (.not. x?=w560:bool)
    n377 = And(x=w264, y=w415) -> (x .and. y?=w578:bool)
    n378 = Not And(1:w560, 2:w257) -> (0:w562:bool)
    n379 = Compound Arithmetic op=AND(w233, w288, w295) -> (w304:bool)
    n380 = Compound Arithmetic op=AND(w294, w288, w292) -> (w303:bool)
    n381 = Compound Arithmetic op=AND(w391, w486, w488, w485) -> (w494:bool)
    n382 = Compound Arithmetic op=AND(w391, w491, w489, w485) -> (w496:bool)
    n383 = Not(x=w304) -> (.not. x?=w290:bool)
    n384 = Not(x=w303) -> (.not. x?=w291:bool)
    n385 = Not(x=w494) -> (.not. x?=w493:bool)
    n386 = Not(x=w496) -> (.not. x?=w495:bool)
    n387 = Not And(1:w562, 2:w431) -> (0:w525:bool)
    n388 = Not(x=w124) -> (.not. x?=w322:bool)
    n389 = Compound Arithmetic op=AND(w288, w288, w285) -> (w289:bool)
    n390 = Compound Arithmetic op=AND(w290, w291, w291) -> (w302:bool)
    n391 = Not(x=w289) -> (.not. x?=w284:bool)
    n392 = And(x=w495, y=w87) -> (x .and. y?=w500:bool)
    n393 = And(x=w85, y=w493) -> (x .and. y?=w498:bool)
    n394 = Not(x=w302) -> (.not. x?=w159:bool)
    "BT" <- w159
    n395 = Compound Arithmetic op=AND(w319, w126, w322) -> (w340:bool)
    n396 = Not(x=w340) -> (.not. x?=w336:bool)
    n397 = Compound Arithmetic op=AND(w52, w422, w181) -> (w548:bool)
    n398 = Compound Arithmetic op=OR(w500, w499, w498, w484) -> (w497:bool)
    n399 = Not And(1:w283, 2:w283) -> (0:w323:bool)
    n400 = Not And(1:w287, 2:w284) -> (0:w286:bool)
    n401 = Not And(1:w285, 2:w286) -> (0:w282:bool)
    "LS" <- w282
    n402 = Compound Arithmetic op=AND(w124, w126, w282) -> (w339:bool)
    n403 = Not(x=w339) -> (.not. x?=w328:bool)
    n404 = feedback-in #35(w282) -> ()
    n405 = Not(x=w548) -> (.not. x?=w547:bool)
    n406 = And(x=w6, y=w264) -> (x .and. y?=w556:bool)
    n407 = And(x=w139, y=w435) -> (x .and. y?=w557:bool)
    n408 = Not(x=w497) -> (.not. x?=w385:bool)
    "R" <- w385
    n409 = Exclusive Or(1:w619, 2:w385) -> (0:w620:bool)
    n410 = Not And(1:w620, 2:w626) -> (0:w623:bool)
    n411 = Not And(1:w606, 2:w623) -> (0:w624:bool)
    n412 = call "DflipFlop.vi"("D"=w624, "Clock"=w621, "Reset"=w622, "Set"=w622) -> ("/Q\\"=w57:bool, "Q"=w625:bool)  [unwired: 6 in]
    n413 = feedback-in #14(w625) -> ()
    n414 = Not And(1:w57, 2:w57) -> (0:w58:bool)
    "CM" <- w58
    n415 = Compound Arithmetic op=AND(w58, w58, w58) -> (w579:bool)
    n416 = Not(x=w579) -> (.not. x?=w549:bool)
    n417 = Not And(1:w58, 2:w564) -> (0:w565:bool)
    n418 = Compound Arithmetic op=AND(w434, w58, w434) -> (w567:bool)
    n419 = Not And(1:w565, 2:w565) -> (0:w563:bool)
    n420 = Not(x=w567) -> (.not. x?=w566:bool)
    n421 = And(x=w490, y=w58) -> (x .and. y?=w580:bool)
    n422 = And(x=w54, y=w563) -> (x .and. y?=w581:bool)
    n423 = And(x=w566, y=w56) -> (x .and. y?=w582:bool)
    n424 = Not And(1:w58, 2:w56) -> (0:w541:bool)
    n425 = Not And(1:w58, 2:w56) -> (0:w569:bool)
    n426 = Compound Arithmetic op=OR(w580, w581, w582, w583) -> (w584:bool)
    n427 = Not And(1:w569, 2:w569) -> (0:w570:bool)
    n428 = Not(x=w584) -> (.not. x?=w535:bool)
    n429 = Compound Arithmetic op=AND(w54, w58, w503) -> (w568:bool)
    n430 = And(x=w573, y=w58) -> (x .and. y?=w577:bool)
    n431 = And(x=w194, y=w570) -> (x .and. y?=w575:bool)
    n432 = Not(x=w568) -> (.not. x?=w528:bool)
    n433 = Compound Arithmetic op=OR(w578, w577, w576, w575) -> (w574:bool)
    n434 = Not(x=w574) -> (.not. x?=w526:bool)
    n435 = Not And(1:w549, 2:w56) -> (0:w550:bool)
    n436 = Compound Arithmetic op=AND(w328, w328, w328) -> (w329:bool)
    n437 = Not And(1:w322, 2:w323) -> (0:w320:bool)
    n438 = Not And(1:w124, 2:w283) -> (0:w144:bool)
    n439 = Not And(1:w336, 2:w336) -> (0:w335:bool)
    n440 = Compound Arithmetic op=OR(w555, w556, w557, w558) -> (w559:bool)
    n441 = Not(x=w329) -> (.not. x?=w327:bool)
    n442 = Compound Arithmetic op=AND(w551, w547, w550) -> (w553:bool)
    n443 = Not(x=w553) -> (.not. x?=w552:bool)
    n444 = Not(x=w559) -> (.not. x?=w518:bool)
    n445 = Compound Arithmetic op=AND(w337, w336, w312) -> (w338:bool)
    n446 = Not And(1:w335, 2:w313) -> (0:w330:bool)
    n447 = Compound Arithmetic op=AND(w144, w320, w319) -> (w321:bool)
    n448 = Not And(1:w319, 2:w327) -> (0:w325:bool)
    n449 = Not And(1:w334, 2:w216) -> (0:w331:bool)
    n450 = Not And(1:w155, 2:w124) -> (0:w235:bool)
    n451 = Not(x=w338) -> (.not. x?=w332:bool)
    n452 = Not(x=w321) -> (.not. x?=w318:bool)
    n453 = Not And(1:w552, 2:w552) -> (0:w517:bool)
    n454 = Not And(1:w325, 2:w314) -> (0:w324:bool)
    n455 = Compound Arithmetic op=AND(w233, w232, w235, w182) -> (w237:bool)
    n456 = Not And(1:w318, 2:w318) -> (0:w315:bool)
    "HF" <- w315
    n457 = Compound Arithmetic op=AND(w332, w331, w330) -> (w333:bool)
    n458 = Not(x=w237) -> (.not. x?=w236:bool)
    n459 = Not And(1:w324, 2:w324) -> (0:w316:bool)
    "JW3" <- w316
    n460 = Not(x=w333) -> (.not. x?=w317:bool)
    "JW7" <- w317
    n461 = call "DflipFlop.vi"("D"=w236, "Clock"=w197, "Reset"=w238, "Set"=w238) -> ("/Q\\"=w28:bool, "Q"=w29:bool)  [unwired: 6 in]
    "TS" <- w28
    n462 = Not And(1:w530, 2:w58) -> (0:w529:bool)
    n463 = Not And(1:w520, 2:w58) -> (0:w516:bool)
    n464 = Not And(1:w227, 2:w227) -> (0:w228:bool)
    n465 = call "7495.vi"("Clk 1\nR-Shift"=w106, "Serial\nInput"=w317, "Clk 2\nL-Shift"=w106, "Mode\nControl"=w315, "D"=w314, "C"=w357, "B"=w356, "A"=w313) -> ("OD"=w349:bool, "OC"=w352:bool, "OB"=w354:bool, "OA"=w355:bool)
    "W4" <- w349
    "W5" <- w352
    "W6" <- w354
    "W7" <- w355
    n466 = feedback-in #37(w355) -> ()
    n467 = feedback-in #38(w354) -> ()
    n468 = feedback-in #39(w352) -> ()
    n469 = feedback-in #40(w349) -> ()
    n470 = Compound Arithmetic op=AND(w227, w280, w181, w279, w280, w143, w194, w190) -> (w281:bool)
    n471 = Not And(1:w143, 2:w143) -> (0:w140:bool)
    n472 = Not And(1:w228, 2:w143) -> (0:w226:bool)
    n473 = Not(x=w281) -> (.not. x?=w278:bool)
    n474 = Not(x=w278) -> (.not. x?=w267:bool)
    "LONGLOGIC" <- w267
    n475 = call "7495.vi"("Clk 1\nR-Shift"=w106, "Serial\nInput"=w316, "Clk 2\nL-Shift"=w106, "Mode\nControl"=w315, "D"=w312, "C"=w358, "B"=w359, "A"=w360) -> ("OD"=w151:bool, "OC"=w350:bool, "OB"=w351:bool, "OA"=w353:bool)
    "W0" <- w151
    "W1" <- w350
    "W2" <- w351
    "W3" <- w353
    n476 = feedback-in #41(w353) -> ()
    n477 = feedback-in #42(w351) -> ()
    n478 = feedback-in #43(w350) -> ()
    n479 = feedback-in #44(w151) -> ()
    n480 = Not And(1:w261, 2:w182) -> (0:w260:bool)
    n481 = Not And(1:w265, 2:w267) -> (0:w258:bool)
    n482 = Not(x=w190) -> (.not. x?=w189:bool)
    n483 = Not And(1:w259, 2:w258) -> (0:w251:bool)
    n484 = Not And(1:w260, 2:w257) -> (0:w253:bool)
    n485 = Not And(1:w258, 2:w177) -> (0:w255:bool)
    n486 = Not And(1:w194, 2:w182) -> (0:w266:bool)
    n487 = Compound Arithmetic op=AND(w255, w255, w255) -> (w277:bool)
    n488 = Not And(1:w163, 2:w163) -> (0:w160:bool)
    n489 = Not(x=w277) -> (.not. x?=w256:bool)
    n490 = Compound Arithmetic op=AND(w160, w159, w158) -> (w161:bool)
    n491 = Not(x=w161) -> (.not. x?=w157:bool)
    n492 = And(x=w87, y=w251) -> (x .and. y?=w273:bool)
    n493 = And(x=w151, y=w253) -> (x .and. y?=w272:bool)
    n494 = Compound Arithmetic op=AND(w151, w255, w255) -> (w275:bool)
    n495 = Not And(1:w157, 2:w157) -> (0:w125:bool)
    "BM" <- w125
    n496 = Not(x=w275) -> (.not. x?=w254:bool)
    n497 = Compound Arithmetic op=AND(w145, w144, w140) -> (w147:bool)
    n498 = And(x=w125, y=w162) -> (x .and. y?=w172:bool)
    n499 = And(x=w152, y=w143) -> (x .and. y?=w165:bool)
    n500 = And(x=w155, y=w125) -> (x .and. y?=w167:bool)
    n501 = Not(x=w147) -> (.not. x?=w142:bool)
    n502 = Compound Arithmetic op=AND(w142, w139, w5) -> (w146:bool)
    n503 = Not(x=w146) -> (.not. x?=w141:bool)
    n504 = Not And(1:w182, 2:w181) -> (0:w180:bool)
    n505 = Not And(1:w180, 2:w104) -> (0:w154:bool)
    "WJ" <- w154
    n506 = And(x=w154, y=w154) -> (x .and. y?=w170:bool)
    n507 = Not And(1:w190, 2:w182) -> (0:w219:bool)
    "ADD" <- w219
    n508 = feedback #48() -> (w132:bool)  [unwired: 1 in]
    n509 = Compound Arithmetic op=AND(w132, w142, w141) -> (w148:bool)
    n510 = Not(x=w148) -> (.not. x?=w136:bool)
    n511 = Compound Arithmetic op=AND(w48, w48, w136) -> (w137:bool)
    n512 = Not(x=w137) -> (.not. x?=w134:bool)
    n513 = call "DflipFlop.vi"("D"=w134, "Clock"=w135, "Reset"=w149, "Set"=w149) -> ("/Q\\"=→"ED":bool, "Q"=w62:bool)  [unwired: 6 in]
    n514 = Not And(1:w62, 2:w592) -> (0:w587:bool)
    n515 = Compound Arithmetic op=AND(w587, w482, w326, w519) -> (w588:bool)
    n516 = Compound Arithmetic op=AND(w478, w481, w482, w587) -> (w593:bool)
    n517 = Not(x=w588) -> (.not. x?=w586:bool)
    n518 = Not(x=w593) -> (.not. x?=w591:bool)
    n519 = Not And(1:w586, 2:w586) -> (0:w524:bool)
    n520 = Not And(1:w591, 2:w591) -> (0:w522:bool)
    n521 = Compound Arithmetic op=AND(w545, w522, w542, w541, w515, w515, w486, w486) -> (w546:bool)
    n522 = Not(x=w546) -> (.not. x?=w504:bool)
    n523 = feedback-in #32(w504) -> ()
    n524 = Compound Arithmetic op=AND(w524, w524, w535, w534, w537, w537, w533, w391) -> (w540:bool)
    n525 = Not(x=w540) -> (.not. x?=w505:bool)
    n526 = feedback-in #31(w505) -> ()
    n527 = Compound Arithmetic op=AND(w523, w522, w526, w525, w524, w177, w522, w523) -> (w527:bool)
    n528 = Not(x=w527) -> (.not. x?=w507:bool)
    n529 = feedback-in #29(w507) -> ()
    n530 = feedback-in #48(w62) -> ()
    n531 = And(x=w210, y=w210) -> (x .and. y?=w214:bool)
    n532 = feedback #49() -> (w209:bool)  [unwired: 1 in]
    n533 = Not And(1:w222, 2:w209) -> (0:w221:bool)
    n534 = call "DflipFlop.vi"("D"=w221, "Clock"=w220, "Reset"=w224, "Set"=w224) -> ("/Q\\"=w16:bool, "Q"=w15:bool)  [unwired: 6 in]
    "C" <- w16
    n535 = Exclusive Or(1:w56, 2:w104) -> (0:w105:bool)
    n536 = feedback #50() -> (w122:bool)  [unwired: 1 in]
    n537 = Exclusive Or(1:w122, 2:TRUE ("x")) -> (0:w120:bool)
    n538 = feedback #51() -> (w118:bool)  [unwired: 1 in]
    n539 = feedback #52() -> (w112:bool)  [unwired: 1 in]
    n540 = Exclusive Or(1:w112, 2:TRUE ("x")) -> (0:w113:bool)
    n541 = Compound Arithmetic op=AND(w113, w110, w109) -> (w114:bool)
    n542 = Not(x=w114) -> (.not. x?=w108:bool)
    n543 = Not(x=w73) -> (.not. x?=w72:bool)
    n544 = Not(x=w71) -> (.not. x?=w70:bool)
    n545 = feedback #53() -> (w65:bool)  [unwired: 1 in]
    n546 = And(x=w65, y=w362) -> (x .and. y?=w367:bool)
    n547 = And(x=w49, y=w65) -> (x .and. y?=w366:bool)
    n548 = And(x=w65, y=w11) -> (x .and. y?=w412:bool)
    n549 = feedback #54() -> (w64:bool)  [unwired: 1 in]
    n550 = And(x=w64, y=w10) -> (x .and. y?=w411:bool)
    n551 = Not Or(1:w411, 2:w412) -> (0:w231:bool)
    n552 = Not And(1:w246, 2:w231) -> (0:w248:bool)
    n553 = Not And(1:w248, 2:w223) -> (0:w247:bool)
    n554 = Not And(1:w231, 2:w231) -> (0:w127:bool)
    "MR" <- w127
    n555 = And(x=w127, y=w47) -> (x .and. y?=w365:bool)
    n556 = Compound Arithmetic op=OR(w368, w367, w366, w365) -> (w364:bool)
    n557 = Not(x=w364) -> (.not. x?=w363:bool)
    n558 = Not And(1:w363, 2:w363) -> (0:w361:bool)
    n559 = call "7495.vi"("Clk 1\nR-Shift"=w106, "Serial\nInput"=w361, "Clk 2\nL-Shift"=w106, "Mode\nControl"=w369, "D"=w373, "C"=w372, "B"=w371, "A"=w370) -> ("OD"=w24:bool, "OC"=w23:bool, "OB"=w22:bool, "OA"=w21:bool)
    "K4" <- w24
    "K5" <- w23
    "K6" <- w22
    "K7" <- w21
    n560 = feedback-in #10(w21) -> ()
    n561 = feedback-in #11(w22) -> ()
    n562 = feedback-in #12(w23) -> ()
    n563 = feedback-in #13(w24) -> ()
    n564 = call "7495.vi"("Clk 1\nR-Shift"=w106, "Serial\nInput"=w24, "Clk 2\nL-Shift"=w106, "Mode\nControl"=w369, "D"=w374, "C"=w375, "B"=w376, "A"=w377) -> ("OD"=w20:bool, "OC"=w19:bool, "OB"=w18:bool, "OA"=w17:bool)
    "K0" <- w20
    "K1" <- w19
    "K2" <- w18
    "K3" <- w17
    n565 = feedback-in #19(w17) -> ()
    n566 = feedback-in #20(w18) -> ()
    n567 = feedback-in #21(w19) -> ()
    n568 = feedback-in #22(w20) -> ()
    n569 = call "DflipFlop.vi"("D"=w247, "Clock"=w220, "Reset"=w249, "Set"=w249) -> ("/Q\\"=w229:bool, "Q"=w230:bool)  [unwired: 6 in]
    "BD" <- w230
    n570 = feedback-in #36(w229) -> ()
    n571 = Compound Arithmetic op=AND(w229, w231, w140) -> (w242:bool)
    n572 = Compound Arithmetic op=AND(w226, w226, w127) -> (w241:bool)
    n573 = Compound Arithmetic op=AND(w227, w231, w230) -> (w244:bool)
    n574 = Not(x=w242) -> (.not. x?=w239:bool)
    n575 = Not(x=w241) -> (.not. x?=w240:bool)
    n576 = Not(x=w244) -> (.not. x?=w243:bool)
    n577 = Compound Arithmetic op=AND(w239, w243, w235, w240) -> (w245:bool)
    n578 = Not(x=w245) -> (.not. x?=w225:bool)
    "JC" <- w225
    n579 = Not And(1:w225, 2:w585) -> (0:w514:bool)
    n580 = Compound Arithmetic op=AND(w523, w514, w528, w479, w529, w485, w440, w109) -> (w532:bool)
    n581 = Not(x=w532) -> (.not. x?=w506:bool)
    n582 = feedback-in #30(w506) -> ()
    n583 = Compound Arithmetic op=AND(w518, w517, w515, w516, w481, w514, w486, w480) -> (w521:bool)
    n584 = Not(x=w521) -> (.not. x?=w60:bool)
    n585 = feedback-in #28(w60) -> ()
    n586 = Not And(1:w127, 2:w194) -> (0:w192:bool)
    n587 = Compound Arithmetic op=AND(w191, w189, w192) -> (w193:bool)
    n588 = Not(x=w193) -> (.not. x?=w188:bool)
    n589 = Compound Arithmetic op=AND(w266, w127, w256) -> (w276:bool)
    n590 = Not And(1:w181, 2:w188) -> (0:w185:bool)
    n591 = Not(x=w276) -> (.not. x?=w269:bool)
    n592 = Not And(1:w185, 2:w182) -> (0:w184:bool)
    n593 = Not And(1:w254, 2:w269) -> (0:w218:bool)
    "A" <- w218
    n594 = Not And(1:w183, 2:w184) -> (0:w9:bool)
    "WK" <- w9
    n595 = And(x=w9, y=w9) -> (x .and. y?=w173:bool)
    n596 = And(x=w9, y=w151) -> (x .and. y?=w164:bool)
    n597 = Compound Arithmetic op=OR(w173, w172, w171, w170) -> (w169:bool)
    n598 = Not(x=w169) -> (.not. x?=w156:bool)
    n599 = Not And(1:w156, 2:w156) -> (0:w94:bool)
    "WT" <- w94
    n600 = Exclusive Or(1:w218, 2:w219) -> (0:w202:bool)
    n601 = Not And(1:w202, 2:w202) -> (0:w205:bool)
    n602 = Exclusive Or(1:w126, 2:w127) -> (0:w128:bool)
    n603 = Compound Arithmetic op=AND(w128, w125, w124) -> (w129:bool)
    n604 = And(x=w15, y=w202) -> (x .and. y?=w211:bool)
    n605 = Not(x=w129) -> (.not. x?=w119:bool)
    "KP" <- w119
    n606 = Not And(1:w119, 2:w118) -> (0:w117:bool)
    n607 = Not And(1:w119, 2:w120) -> (0:w123:bool)
    n608 = Not And(1:w116, 2:w117) -> (0:w115:bool)
    n609 = call "7495.vi"("Clk 1\nR-Shift"=w106, "Serial\nInput"=w107, "Clk 2\nL-Shift"=w106, "Mode\nControl"=w105, "D"=w108, "C"=w115, "B"=w123, "A"=w107) -> ("OD"=w103:bool, "OC"=w130:bool, "OB"=w131:bool)  [unwired: 1 out]
    "PO" <- w103
    "PT" <- w130
    "PF" <- w131
    n610 = And(x=w252, y=w103) -> (x .and. y?=w274:bool)
    n611 = Compound Arithmetic op=OR(w274, w273, w272, w271) -> (w270:bool)
    n612 = Not(x=w270) -> (.not. x?=w203:bool)
    "B" <- w203
    n613 = Not And(1:w203, 2:w203) -> (0:w204:bool)
    n614 = Exclusive Or(1:w203, 2:w218) -> (0:w217:bool)
    n615 = Exclusive Or(1:w15, 2:w217) -> (0:w153:bool)
    "SUM" <- w153
    n616 = And(x=w154, y=w153) -> (x .and. y?=w166:bool)
    n617 = Compound Arithmetic op=OR(w164, w165, w166, w167) -> (w168:bool)
    n618 = Not(x=w168) -> (.not. x?=w150:bool)
    n619 = Not And(1:w150, 2:w150) -> (0:w96:bool)
    "WD" <- w96
    n620 = feedback-in #47(w153) -> ()
    n621 = Compound Arithmetic op=AND(w205, w204, w15) -> (w208:bool)
    n622 = Compound Arithmetic op=AND(w202, w203, w16) -> (w207:bool)
    n623 = Not(x=w208) -> (.not. x?=w200:bool)
    n624 = Not(x=w207) -> (.not. x?=w201:bool)
    n625 = Compound Arithmetic op=AND(w200, w200, w201) -> (w206:bool)
    n626 = And(x=w203, y=w202) -> (x .and. y?=w212:bool)
    n627 = And(x=w203, y=w15) -> (x .and. y?=w213:bool)
    n628 = Not(x=w206) -> (.not. x?=w196:bool)
    "OF" <- w196
    n629 = call "DflipFlop.vi"("D"=w196, "Clock"=w197, "Reset"=w199, "Set"=w199) -> ("Q"=w86:bool)  [unwired: 6 in, 1 out]
    "OV" <- w86
    n630 = Compound Arithmetic op=OR(w211, w212, w213, w214) -> (w215:bool)
    n631 = Not(x=w215) -> (.not. x?=w195:bool)
    "CR" <- w195
    n632 = call "DflipFlop.vi"("D"=w195, "Clock"=w197, "Reset"=w198, "Set"=w198) -> ("Q"=w84:bool)  [unwired: 6 in, 1 out]
    "CY" <- w84
    n633 = feedback-in #49(w195) -> ()
    n634 = feedback-in #50(w131) -> ()
    n635 = feedback-in #51(w130) -> ()
    n636 = feedback-in #52(w103) -> ()
    n637 = Not And(1:w86, 2:w87) -> (0:w89:bool)
    n638 = Not And(1:w84, 2:w85) -> (0:w88:bool)
    n639 = Not And(1:w10, 2:w94) -> (0:w99:bool)
    n640 = Not And(1:w11, 2:w94) -> (0:w91:bool)
    n641 = Not And(1:w88, 2:w89) -> (0:w90:bool)
    n642 = Not And(1:w90, 2:w28) -> (0:w83:bool)
    n643 = Not And(1:w99, 2:w99) -> (0:w102:bool)
    n644 = Not And(1:w91, 2:w91) -> (0:w95:bool)
    n645 = Compound Arithmetic op=AND(w29, w65, w91, w79) -> (w93:bool)
    n646 = Not And(1:w96, 2:w102) -> (0:w101:bool)
    n647 = Not And(1:w64, 2:w99) -> (0:w100:bool)
    n648 = Not(x=w93) -> (.not. x?=w92:bool)
    n649 = Not And(1:w96, 2:w95) -> (0:w97:bool)
    n650 = Not And(1:w100, 2:w101) -> (0:w1:bool)
    "JDL0" <- w1
    n651 = Compound Arithmetic op=AND(w92, w83, w97, w77) -> (w98:bool)
    n652 = Not(x=w98) -> (.not. x?=w75:bool)
    "JDL1" <- w75
    n653 = Not And(1:w1, 2:w1) -> (0:w76:bool)
    n654 = Not And(1:w75, 2:w75) -> (0:w74:bool)
    n655 = call "Mem1024.vi"("Phi2"=w70, "Phi1"=w72, "Data In"=w76) -> ("Data Out"=w3:bool)  [unwired: 8 in]
    n656 = call "Mem1024.vi"("Phi2"=w70, "Phi1"=w72, "Data In"=w74) -> ("Data Out"=w69:bool)  [unwired: 8 in]
    n657 = call "Mem2Num.vi"("Data In"=w1) -> ("Mem"=→"mem":u8)  [unwired: 10 in]
    n658 = Not And(1:w3, 2:w68) -> (0:w67:bool)
    n659 = feedback-in #54(w67) -> ()
    n660 = Not And(1:w69, 2:w68) -> (0:w66:bool)
    n661 = feedback-in #53(w66) -> ()
  }
